vi "one_consumer.vi"() -> ()   [LabVIEW 2020]
uses:
  Type Defs/Message.ctl
panel:
  in  "b":bool
  in  "a":bool
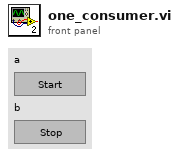
[diagram p1: front panel]
types:
  T1 = typedef "Message.ctl" = cluster{"Command":string, "Data":variant}
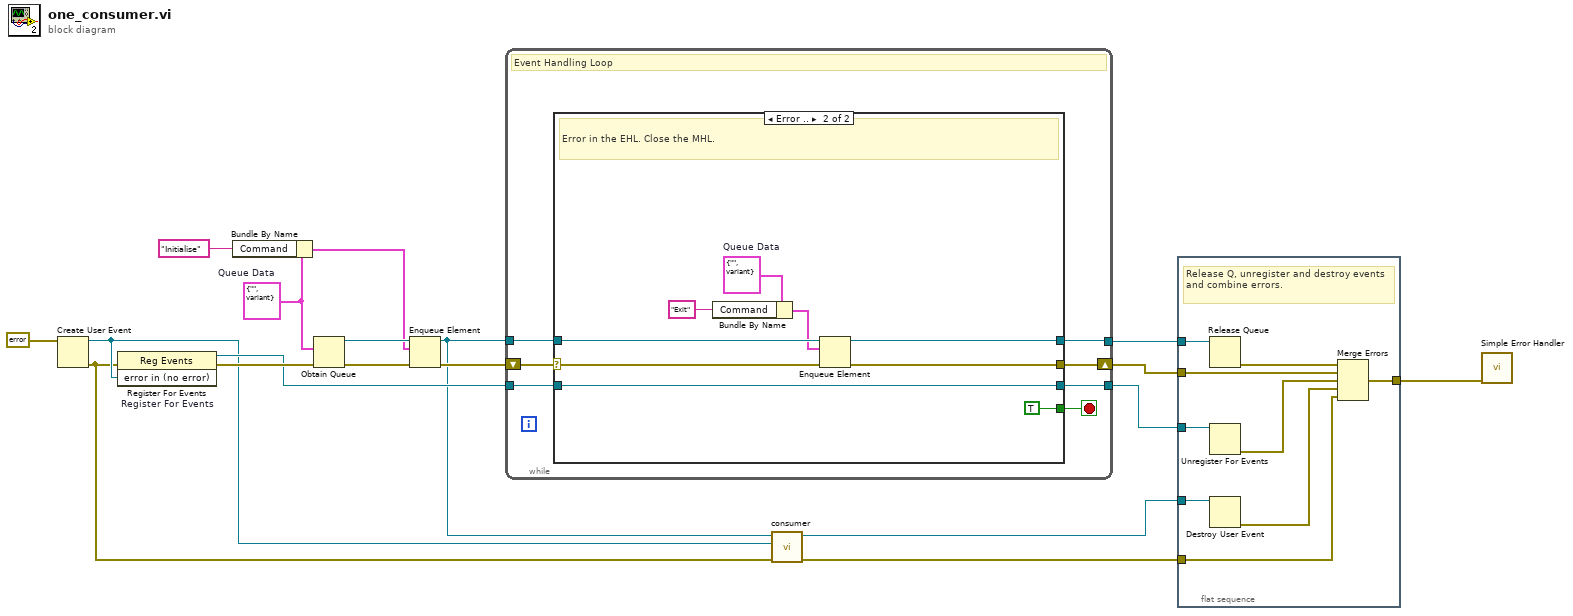
[diagram p0: block diagram]
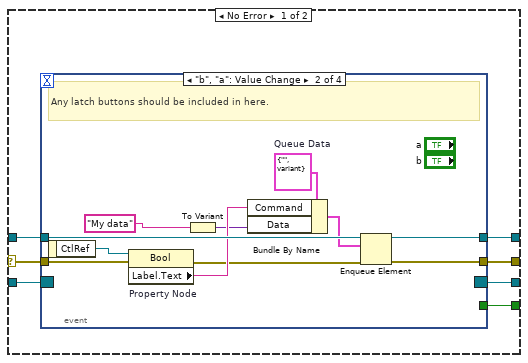
[diagram p2: hidden frame]
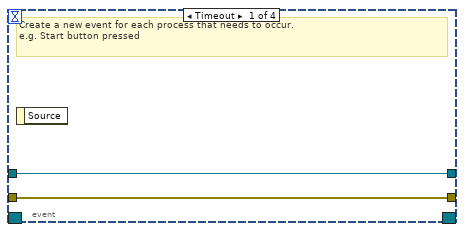
[diagram p3: hidden frame]
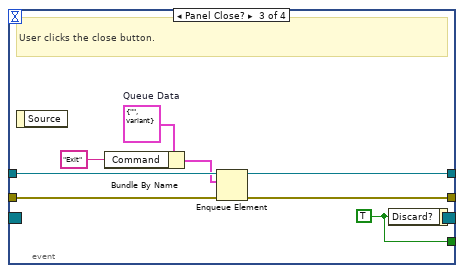
[diagram p4: hidden frame]
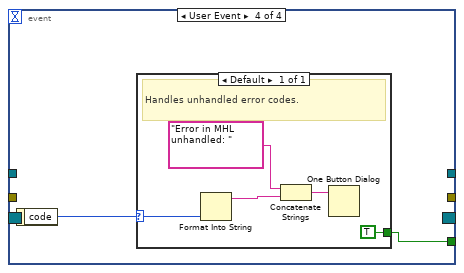
[diagram p5: hidden frame]
diagram:
  w4 = T1 {"Command"="", "Data"=variant}  # Queue Data
  n1 = Create User Event(user event datatype=errorcluster {"status"=FALSE, "code"=0, "source"=""} ("error in (no error)")) -> (user event=w15:refnum<user-event>, error out=w14:errorcluster)  [unwired: 1 in]
  n2 = register-events "Register For Events"(error in=w14, w15) -> (reference out=w16:refnum<event-registration>, error out=w17:errorcluster)  [unwired: 1 in]
  n3 = Bundle By Name "Bundle By Name"(cluster=w4, "Command"="Initialise") -> (w5:T1)
  n4 = Obtain Queue(element data type=w4, error in (no error)=w17) -> (queue out=w9:refnum<queue>, error out=w8:errorcluster)  [unwired: 3 in, 1 out]
  n5 = Enqueue Element(queue=w9, element=w5, error in (no error)=w8) -> (queue out=w6:refnum<queue>, error out=w7:errorcluster)  [unwired: 1 in, 1 out]
  n6 = while {
    tunnel: w6 -> [w24]
    shift-right: [w25] -> w2
    shift-left: w7 -> [w19]
    tunnel: [w23] -> w18
    tunnel: w16 -> [w22]
    tunnel: [w21] -> w13
    stop <- w20 stop-if-true
    # "Event Handling Loop"
    n7 = case shown="Error .." w19 {
      selector: w19 -> [w26 w67]
      tunnel: [w32 w66] -> w25
      tunnel: w24 -> [w31 w64]
      tunnel: [w30 w65] -> w23
      tunnel: w22 -> [w29 w69]
      tunnel: [w28 w69] -> w21
      tunnel: [w27 TRUE ("Stop Event")] -> w20
      frame No Error {
        n8 = event shown="[1] \"b\", \"a\": Value Change" {
          selector: w29 -> [_ _ _ _]
          dyn-events: [_ _ _ _] -> w28
          timeout: _ -> [_ _ _ _]
          tunnel: w26 -> [w34 w38 w53 _]
          tunnel: [w34 w45 w50 _] -> w32
          tunnel: w31 -> [w33 w44 w52 _]
          tunnel: [w33 w43 w51 _] -> w30
          tunnel: [_ _ w46 w54] -> w27
          event Timeout {
            # "Create a new event for each process that needs to occur. \ne.g. Start button pressed"
            n9 = event-data() -> ()  [unwired: 1 in, 1 out]
          }
          event "b", "a": Value Change {
            w42 = T1 {"Command"="", "Data"=variant}  # Queue Data
            # "Any latch buttons should be included in here."
            n10 = event-data() -> ("CtlRef"=w40:refnum<vi>)  [unwired: 1 in]
            n11 = property on="Property Node" class="Bool"(reference=w40, error in=w38) -> (error out=w37:errorcluster, "Label.Text"=w39:string)  [unwired: 1 out]
            n12 = To Variant(anything="My data") -> (Variant=w35:variant)
            n13 = Bundle By Name(cluster=w42, "Command"=w39, "Data"=w35) -> (w41:T1)
            n14 = Enqueue Element(queue=w44, element=w41, error in (no error)=w37) -> (queue out=w43:refnum<queue>, error out=w45:errorcluster)  [unwired: 1 in, 1 out]
          }
          event Panel Close? {
            w49 = T1 {"Command"="", "Data"=variant}  # Queue Data
            w46 = TRUE ("Discard?")
            # "User clicks the close button."
            n15 = event-data() -> ()  [unwired: 1 in, 1 out]
            n16 = Bundle By Name(cluster=w49, "Command"="Exit") -> (w47:T1)
            n17 = Enqueue Element(queue=w52, element=w47, error in (no error)=w53) -> (queue out=w51:refnum<queue>, error out=w50:errorcluster)  [unwired: 1 in, 1 out]
            n18 = event-data("Discard?"=w46) -> ()  [unwired: 1 in, 1 out]
          }
          event User Event {
            n19 = event-data() -> ("code"=w55:i32)  [unwired: 1 in]
            n20 = case shown="Default" w55 {
              selector: w55 -> [w57]
              tunnel: [TRUE] -> w54
              frame Default {
                # "Handles unhandled error codes."
                n21 = Format Into String(w57) -> (resulting string=w58:string)  [unwired: 3 in, 1 out]
                n22 = Concatenate Strings("Error in MHL unhandled: ", w58) -> (w60:string)
                n23 = One Button Dialog(message=w60) -> ()  [unwired: 1 in, 1 out]
              }
            }
          }
        }
      }
      frame Error {
        w63 = T1 {"Command"="", "Data"=variant}  # Queue Data
        # "Error in the EHL. Close the MHL."
        n24 = Bundle By Name(cluster=w63, "Command"="Exit") -> (w62:T1)
        n25 = Enqueue Element(queue=w64, element=w62, error in (no error)=w67) -> (queue out=w65:refnum<queue>, error out=w66:errorcluster)  [unwired: 1 in, 1 out]
      }
    }
  }
  n26 = call "consumer.vi"("error in (no error)"=w14, "user event in"=w15, "Queue in"=w6) -> ("error out"=w11:errorcluster, "user event out"=w12:refnum<user-event>)  [unwired: 7 in]
  n27 = flat-sequence {
    tunnel: w18 -> [w78]
    tunnel: w13 -> [w77]
    tunnel: w12 -> [w76]
    tunnel: w11 -> [w75]
    tunnel: [w74] -> w10
    tunnel: w2 -> [w70]
    frame #0 {
      # "Release Q, unregister and destroy events and combine errors."
      n28 = Release Queue(queue=w78) -> (error out=w71:errorcluster)  [unwired: 2 in, 2 out]
      n29 = Unregister For Events(event registration refnum=w77) -> (error out=w72:errorcluster)  [unwired: 1 in]
      n30 = Destroy User Event(user event=w76) -> (error out=w73:errorcluster)  [unwired: 1 in]
      n31 = Merge Errors(w71, w70, w72, w73, w75) -> (w74:errorcluster)
    }
  }
  n32 = call <vilib>:"Simple Error Handler.vi"("error in (no error)"=w10) -> ()  [unwired: 4 in, 5 out]
